vi "FTW-CodeGen-GenerateCode.vi"(0 "State In":T2, 5 "XRef":refnum<vi>, 7 "Terms":T1(array[cluster]), 9 "Diagram":refnum<vi>) -> (4 "State Out":T2, 6 "Reply":string[](array[string]), 8 "Generated Code?":bool)   [LabVIEW 2015, in "FTW-dotNet-MySQL-Fetch.xnode"]
uses:
  FTW-dotNet-MySQL-Fetch.xnode
  FTW-CodeGen-State.ctl
  src/reflection/FTW-Reflection-Types.ctl
panel:
  # "Inputs"
  # "Outputs"
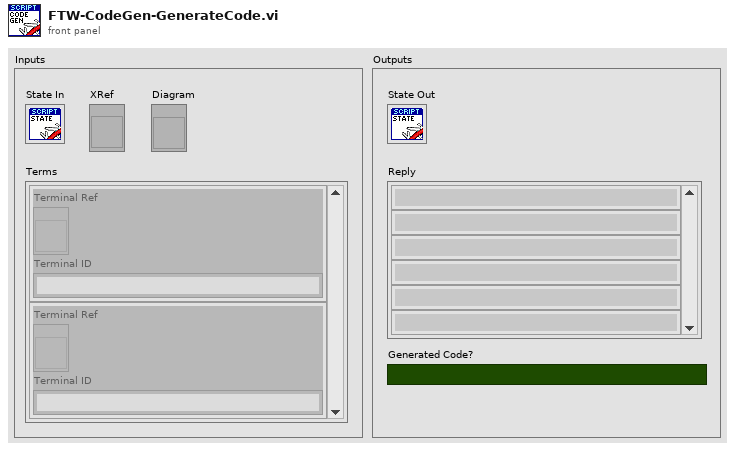
[diagram p1: front panel]
types:
  T1 = cluster{"Terminal Ref":refnum<vi>, "Terminal ID":string}[]
  T2 = typedef "FTW-dotNet-MySQL-Fetch.xnode/FTW-CodeGen-State.ctl" = cluster{"Dummy":string}
  T3 = typedef "LVPositionTypeDef.ctl" = cluster{"Left":i32, "Top":i32}
  T4 = typedef "FTW-Reflection-Types.ctl" = enum16{"Unknown", "Void", "Array", "Cluster", "LVObject", "Boolean", "I8", "I16", "I32", "I64", "U8", "U16", "U32", "U64", "SGL", "DBL", "EXT", "CSG", "CDB", "CXT", "FXP", "EnumU8", "EnumU16", "EnumU32", "EnumU64", "SGLwithUnit", "DBLwithUnit", "EXTwithUnit", "CSGwithUnit", "CDBwithUnit", "CXTwithUnit", "String", "Path", "Picture", "Tag", "LVVariant", "Timestamp", "WaveformI8", "WaveformI16", "WaveformI32", "WaveformI64", "WaveformU8", "WaveformU16", "WaveformU32", "WaveformU64", "WaveformSGL", "WaveformDBL", "WaveformEXT", "WaveformCSG", "WaveformCDB", "WaveformCXT", "WaveformDigital", "WaveformUnknownType", "DigitalData", "DynamicData", "ExternalData", "FileByteStream", "TDMStream", "dotNET", "ActiveX", "VIServerReference", "VIReference", "ApplicationInstance", "Menu", "ConnectionDataSocket", "ConnectionVISA", "ConnectionBluetooth", "ConnectionIrDA", "ConnectionTCP", "ConnectionUDP", "ConnectionHTTPClient", "ConnectionFTP", "Occurrence", "Notifier", "Queue", "Rendezvous", "Semaphore", "RTFIFO", "EventPublisher", "EventRegistration", "EventCallback", "DataValueReference", "GenericClass", "GenericClassTag", "GenericClassDeepCopy", "GenericClassFlattened", "GenericClassTagFlattened", "GenericReferenceType", "WindowsRegistry", "OverloadedDatalogRef", "ReferenceUnknownType", "ByteArray", "ConPaneInterface", "FTWObject"}
  T5 = cluster{"Element Name":string, "Element Type":T4, "Element Value":variant}
  T6 = cluster{"Element Name":string, "Element Type":T4, "Element Value":variant}[]
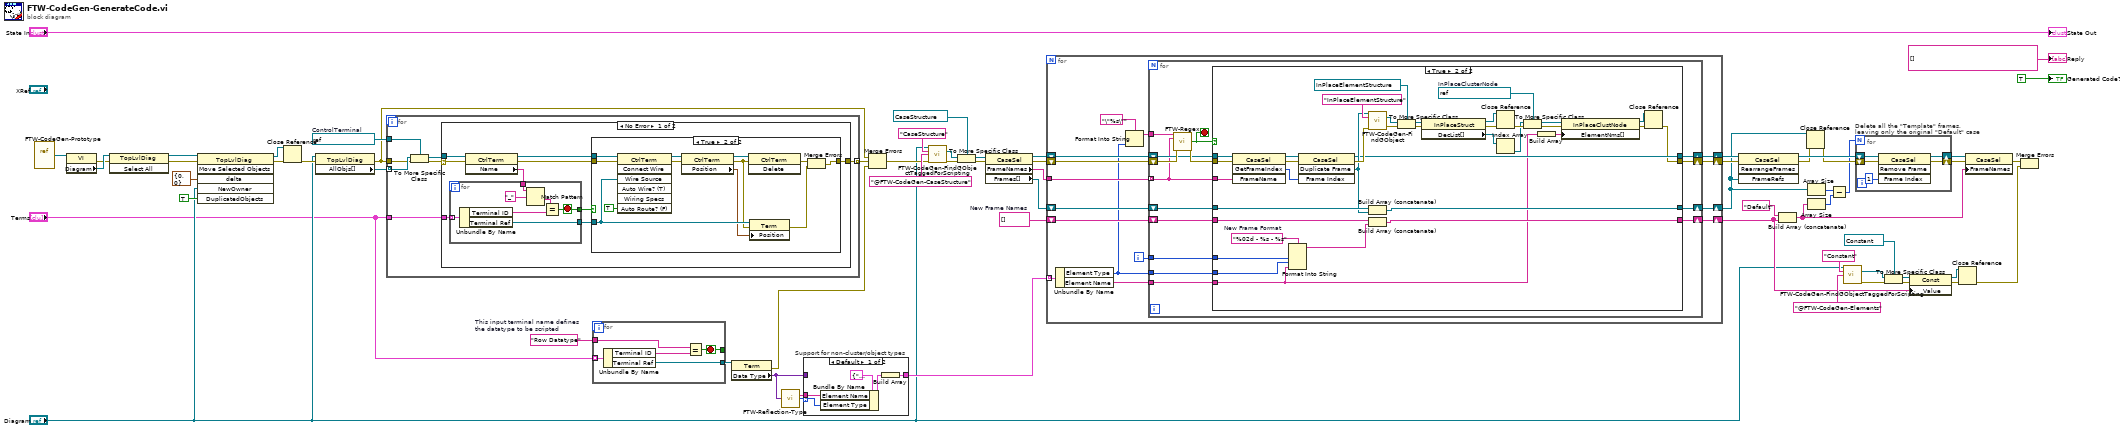
[diagram p0: block diagram]
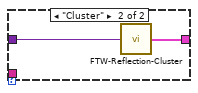
[diagram p2: hidden frame]
diagram:
  w28 = string[] []  # New Frame Names
  w44 = "Row Datatype"  # This input terminal name defines the datatype to be scripted
  w59 = refnum<vi> refnum  # ControlTerminal
  n1 = vi-ref "FTW-CodeGen-Prototype.vi"() -> (w5:refnum<vi>)
  n2 = property class="VI"(reference=w5) -> (error out=w54:errorcluster, "Diagram"=w58:refnum<vi>)  [unwired: 1 in, 1 out]
  n3 = invoke class="TopLvlDiag" method="Select All"(reference=w58, error in=w54) -> (reference out=w62:refnum<vi>, error out=w61:errorcluster)  [unwired: 1 in, 1 out]
  n4 = invoke class="TopLvlDiag" method="Move Selected Objects"(reference=w62, error in=w61, "delta"=cluster{"X":i32, "Y":i32} {"X"=0, "Y"=0} ("X/Y Delta"), "NewOwner"="Diagram", "DuplicatedObjects"=TRUE ("Duplicate? (F)")) -> (reference out=w51:refnum<vi>, error out=w53:errorcluster)  [unwired: 1 in, 4 out]
  n5 = Close Reference(reference=w51, error in (no error)=w53) -> (error out=w52:errorcluster)
  n6 = property class="TopLvlDiag"(reference="Diagram", error in=w52) -> (error out=w56:errorcluster, "AllObjs[]"=w60:refnum<vi>[])  [unwired: 1 out]
  n7 = for {
    tunnel: w60 -> [w71] mode=indexing
    tunnel: w56 -> [w70]
    tunnel: w59 -> [w69]
    tunnel: "Terms" -> [w66]
    tunnel: [w65] -> w57 mode=indexing
    n8 = To More Specific Class(target class=w69, reference=w71, error in=w70) -> (specific class reference=w67:refnum<vi>, error out=w68:errorcluster)
    n9 = case shown="No Error" w68 {
      selector: w68 -> [w79 _]
      tunnel: w67 -> [w80 _]
      tunnel: w66 -> [w78 _]
      tunnel: [w73 _] -> w65
      frame No Error {
        n10 = property class="CtrlTerm"(reference=w80, error in=w79) -> (reference out=w75:refnum<vi>, error out=w74:errorcluster, "Name"=w77:string)
        n11 = for {
          tunnel: w78 -> [w100] mode=indexing
          tunnel: w77 -> [w98]
          tunnel: [w99] -> w76
          tunnel: [w94] -> w72
          stop <- w94 stop-if-true
          n12 = Unbundle By Name(w100) -> ("Terminal ID"=w95:string, "Terminal Ref"=w99:refnum<vi>)
          n13 = Match Pattern(string=w98, regular expression="_") -> (after substring=w96:string)  [unwired: 1 in, 3 out]
          n14 = Equal?(x=w96, y=w95) -> (x = y?=w94:bool)
        }
        n15 = case shown="True" w72 {
          tunnel: w76 -> [_ w85]
          tunnel: w75 -> [_ w93]
          tunnel: w74 -> [w81 w92]
          tunnel: [w81 w87] -> w73
          frame False {
          }
          frame True {
            n16 = invoke class="CtrlTerm" method="Connect Wire"(reference=w93, error in=w92, "Wire Source"=w85, "Auto Route? (F)"=TRUE) -> (reference out=w91:refnum<vi>, error out=w89:errorcluster)  [unwired: 3 in, 5 out]
            n17 = property class="CtrlTerm"(reference=w91, error in=w89) -> (reference out=w90:refnum<vi>, error out=w84:errorcluster, "Position"=w82:T3)
            n18 = invoke class="CtrlTerm" method="Delete"(reference=w90, error in=w84) -> (error out=w88:errorcluster)  [unwired: 1 in, 2 out]
            n19 = property class="Term"(reference=w85, error in=w84, "Position"=w82) -> (error out=w83:errorcluster)  [unwired: 1 out]
            n20 = Merge Errors(w88, w83) -> (w87:errorcluster)
          }
        }
      }
      frame Error {
      }
    }
  }
  n21 = for {
    tunnel: "Terms" -> [w105] mode=indexing
    tunnel: [w104] -> w38
    tunnel: [w102] -> _
    tunnel: w44 -> [w101]
    stop <- w102 stop-if-true
    n22 = Unbundle By Name(w105) -> ("Terminal ID"=w103:string, "Terminal Ref"=w104:refnum<vi>)
    n23 = Equal?(x=w101, y=w103) -> (x = y?=w102:bool)
  }
  n24 = property class="Term"(reference=w38) -> (error out=w8:errorcluster, "Data Type"=w7:variant)  [unwired: 1 in, 1 out]
  n25 = call "FTW-Reflection-Type.vi"("Anything"=w7) -> ("Data Name"=w6:string, "LabVIEW Type"=w9:T4)  [unwired: 12 in, 1 out]
  n26 = case "Support for non-cluster/object types" shown="Default" w9 {
    selector: w9 -> [w106 _]
    tunnel: [w110 w112] -> w37
    tunnel: w7 -> [_ w111]
    tunnel: w6 -> [w107 _]
    frame Default {
      n27 = Bundle By Name(cluster=T5 {"Element Name"="", "Element Type"=enum."Unknown", "Element Value"=variant} ("Element"), "Element Name"=w107, "Element Type"=w106) -> (w108:T5)
      n28 = Build Array(w108) -> (w110:T6)
    }
    frame "Cluster" {
      n29 = call "FTW-Reflection-Cluster.vi"("Cluster"=w111) -> ("Cluster Elements"=w112:T6)  [unwired: 14 in]
    }
  }
  n30 = Merge Errors(w56, w57, w8) -> (w48:errorcluster)
  n31 = call "FTW-CodeGen-FindGObjectTaggedForScripting.vi"("GObject to Traverse"="Diagram", "Class Name"="CaseStructure", "Label Prefix to uniquely identify node"="@FTW-CodeGen-CaseStructure" ("Label to uniquely identify node"), "error in"=w48) -> ("GObject"=w47:refnum<vi>, "error out"=w46:errorcluster)  [unwired: 9 in, 1 out]
  n32 = To More Specific Class(target class=refnum<vi> refnum ("Object"), reference=w47, error in=w46) -> (specific class reference=w36:refnum<vi>, error out=w34:errorcluster)
  n33 = property class="CaseSel"(reference=w36, error in=w34) -> (reference out=w35:refnum<vi>, error out=w33:errorcluster, "FrameNames"=w32:string[], "Frames[]"=w19:refnum<vi>[])
  n34 = for {
    tunnel: w37 -> [w124] mode=indexing
    tunnel: w32 -> [w125]
    shift-right: [w120] -> w24
    shift-left: w35 -> [w127]
    shift-right: [w121] -> w22
    shift-left: w33 -> [w126]
    shift-right: [w119] -> w18
    shift-left: w19 -> [w122]
    shift-right: [w117] -> w25
    shift-left: w28 -> [w118]
    i -> [w114]
    n35 = Unbundle By Name(w124) -> ("Element Type"=w115:T4, "Element Name"=w116:string)
    n36 = Format Into String(format string="\"%s\"", w115) -> (resulting string=w123:string)  [unwired: 2 in, 1 out]
    n37 = for {
      tunnel: w125 -> [w131] mode=indexing
      tunnel: w123 -> [w141]
      shift-right: [w135] -> w120
      shift-left: w127 -> [w139]
      shift-right: [w137] -> w119
      shift-left: w122 -> [w138]
      shift-right: [w136] -> w121
      shift-left: w126 -> [w142]
      shift-right: [w132] -> w117
      shift-left: w118 -> [w133]
      tunnel: w116 -> [w130]
      tunnel: w115 -> [w129]
      tunnel: w114 -> [w128]
      stop <- w134 stop-if-true
      n38 = call "FTW-Regex.vi"("Regular Expression"=w141, "Input String"=w131, "error in"=w142) -> ("Match Found?"=w134:bool, "error out"=w140:errorcluster)  [unwired: 8 in, 3 out]
      n39 = case shown="True" w134 {
        tunnel: w140 -> [w145 w177]
        tunnel: w139 -> [w146 w178]
        tunnel: w138 -> [w144 w182]
        tunnel: [w144 w179] -> w137
        tunnel: [w145 w153] -> w136
        tunnel: [w146 w157] -> w135
        tunnel: w133 -> [w143 w181]
        tunnel: [w143 w180] -> w132
        tunnel: w131 -> [_ w173]
        tunnel: w130 -> [_ w149]
        tunnel: w129 -> [_ w148]
        tunnel: w128 -> [_ w147]
        frame False {
        }
        frame True {
          w150 = "%02d - %s - %s"  # New Frame Format
          w168 = refnum<vi> refnum  # InPlaceClusterNode
          n40 = invoke class="CaseSel" method="GetFrameIndex"(reference=w178, error in=w177, "FrameName"=w173) -> (reference out=w176:refnum<vi>, error out=w175:errorcluster, "GetFrameIndex"=w174:i32)  [unwired: 1 in, 1 out]
          n41 = Format Into String(format string=w150, w147, w148, w149) -> (resulting string=w151:string)  [unwired: 2 in, 1 out]
          n42 = invoke class="CaseSel" method="Duplicate Frame"(reference=w176, error in=w175, "Frame Index"=w174) -> (reference out=w157:refnum<vi>, error out=w159:errorcluster, "Duplicate Frame"=w158:refnum<vi>)  [unwired: 1 in, 1 out]
          n43 = call "FTW-CodeGen-FindGObject.vi"("GObject to Traverse"=w158, "Class Name"="InPlaceElementStructure", "error in"=w159) -> ("GObject"=w161:refnum<vi>, "error out"=w162:errorcluster)  [unwired: 11 in]
          n44 = Build Array (concatenate)(w182, w158) -> (w179:refnum<vi>[])
          n45 = Build Array (concatenate)(w181, w151) -> (w180:string[])
          n46 = To More Specific Class(target class=refnum<vi> refnum ("Object"), reference=w161, error in=w162) -> (specific class reference=w165:refnum<vi>, error out=w164:errorcluster)
          n47 = property class="InPlaceStruct"(reference=w165, error in=w164) -> (reference out=w171:refnum<vi>, error out=w170:errorcluster, "DecList[]"=w166:refnum<vi>[])
          n48 = Close Reference(reference=w171, error in (no error)=w170) -> (error out=w172:errorcluster)
          n49 = Index Array(array=w166) -> (element=w167:refnum<vi>)  [unwired: 1 in]
          n50 = To More Specific Class(target class=w168, reference=w167, error in=w172) -> (specific class reference=w169:refnum<vi>, error out=w156:errorcluster)
          n51 = Build Array(w149) -> (w152:string[])
          n52 = property class="InPlaceClustNode"(reference=w169, error in=w156, "ElementNms[]"=w152) -> (reference out=w155:refnum<vi>, error out=w154:errorcluster)
          n53 = Close Reference(reference=w155, error in (no error)=w154) -> (error out=w153:errorcluster)
        }
      }
    }
  }
  n54 = invoke class="CaseSel" method="RearrangeFrames"(reference=w24, error in=w22, "FrameRefs"=w18) -> (reference out=w23:refnum<vi>, error out=w21:errorcluster)  [unwired: 1 in, 2 out]
  n55 = Build Array (concatenate)("Default", w25) -> (w17:string[])
  n56 = Close Reference(reference=w18, error in (no error)=w21) -> (error out=w20:errorcluster)
  n57 = Array Size(array=w18) -> (size(s)=w16:i32)
  n58 = Array Size(array=w17) -> (size(s)=w15:i32)
  n59 = Subtract(x=w16, y=w15) -> (x-y=w14:i32)
  n60 = call "FTW-CodeGen-FindGObjectTaggedForScripting.vi"("GObject to Traverse"="Diagram", "Class Name"="Constant", "Label Prefix to uniquely identify node"="@FTW-CodeGen-Elements" ("Label to uniquely identify node")) -> ("GObject"=w42:refnum<vi>, "error out"=w41:errorcluster)  [unwired: 10 in, 1 out]
  n61 = for "Delete all the \"Template\" frames,\nleaving only the original \"Default\" case" {
    N: w14 -> [_]
    shift-right: [w184] -> w30
    shift-left: w20 -> [w185]
    shift-right: [w186] -> w31
    shift-left: w23 -> [w187]
    n62 = invoke class="CaseSel" method="Remove Frame"(reference=w187, error in=w185, "Frame Index"=u32 1) -> (reference out=w186:refnum<vi>, error out=w184:errorcluster)  [unwired: 1 in, 2 out]
  }
  n63 = To More Specific Class(target class=refnum<vi> refnum ("Object"), reference=w42, error in=w41) -> (specific class reference=w40:refnum<vi>, error out=w39:errorcluster)
  n64 = property class="Const"(reference=w40, error in=w39, "Value"=w25) -> (reference out=w13:refnum<vi>, error out=w12:errorcluster)
  n65 = Close Reference(reference=w13, error in (no error)=w12) -> (error out=w10:errorcluster)
  n66 = property class="CaseSel"(reference=w31, error in=w30, "FrameNames"=w17) -> (error out=w11:errorcluster)  [unwired: 1 out]
  n67 = Merge Errors(w11, w10) -> ()  [unwired: 1 out]
  "State Out" <- "State In"
  "Reply" <- string[] [] ("Reply")
  "Generated Code?" <- TRUE ("Generated Code?")
